vi "Element List to Scoring Cluster.vi"(11 "Array":cluster{"Name":string, "Value":string}[](array[cluster])) -> (0 "error out":errorcluster, 3 "output cluster":T1)   [LabVIEW 2013]
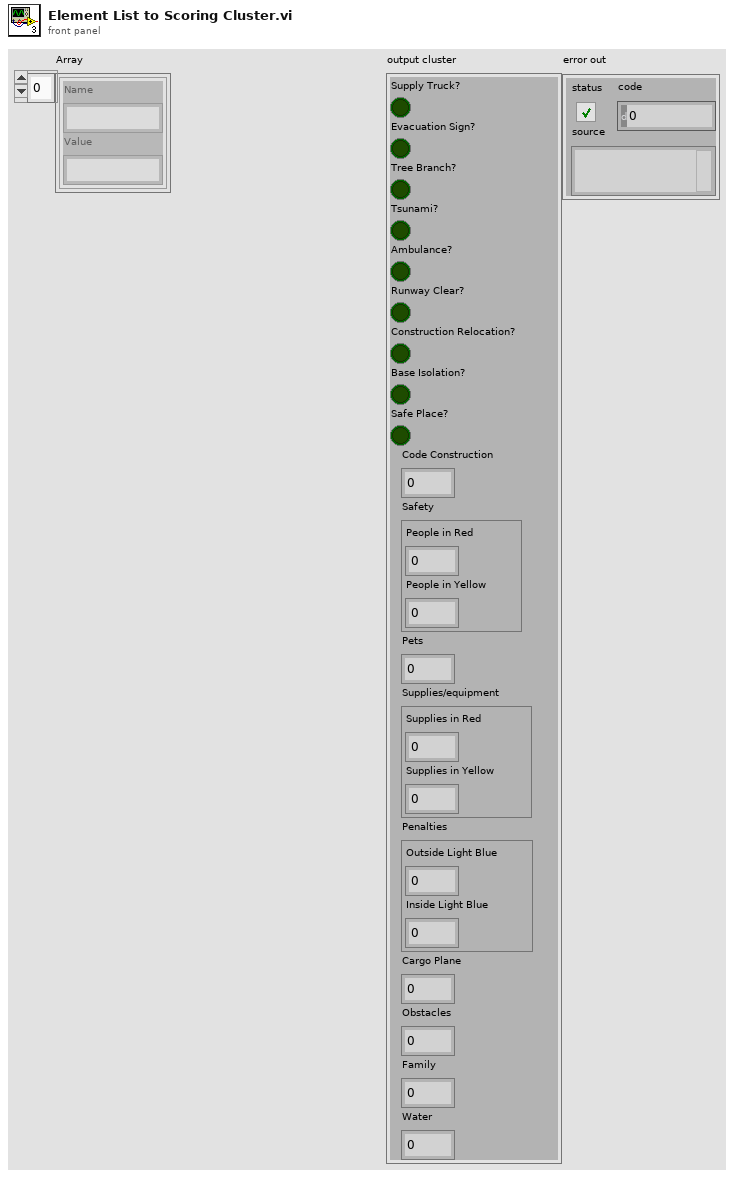
[diagram p1: front panel]
types:
  T1 = cluster{"Supply Truck?":bool, "Evacuation Sign?":bool, "Tree Branch?":bool, "Tsunami?":bool, "Ambulance?":bool, "Runway Clear?":bool, "Construction Relocation?":bool, "Base Isolation?":bool, "Safe Place?":bool, "Code Construction":dbl, "Safety":cluster{"People in Red":dbl, "People in Yellow":dbl}, "Pets":dbl, "Supplies/equipment":cluster{"Supplies in Red":dbl, "Supplies in Yellow":dbl}, "Penalties":cluster{"Outside Light Blue":dbl, "Inside Light Blue":dbl}, "Cargo Plane":u16, "Obstacles":u16, "Family":u16, "Water":dbl}
  T2 = cluster{"People in Red":dbl, "People in Yellow":dbl}
  T3 = cluster{"Outside Light Blue":dbl, "Inside Light Blue":dbl}
  T4 = cluster{"Supplies in Red":dbl, "Supplies in Yellow":dbl}
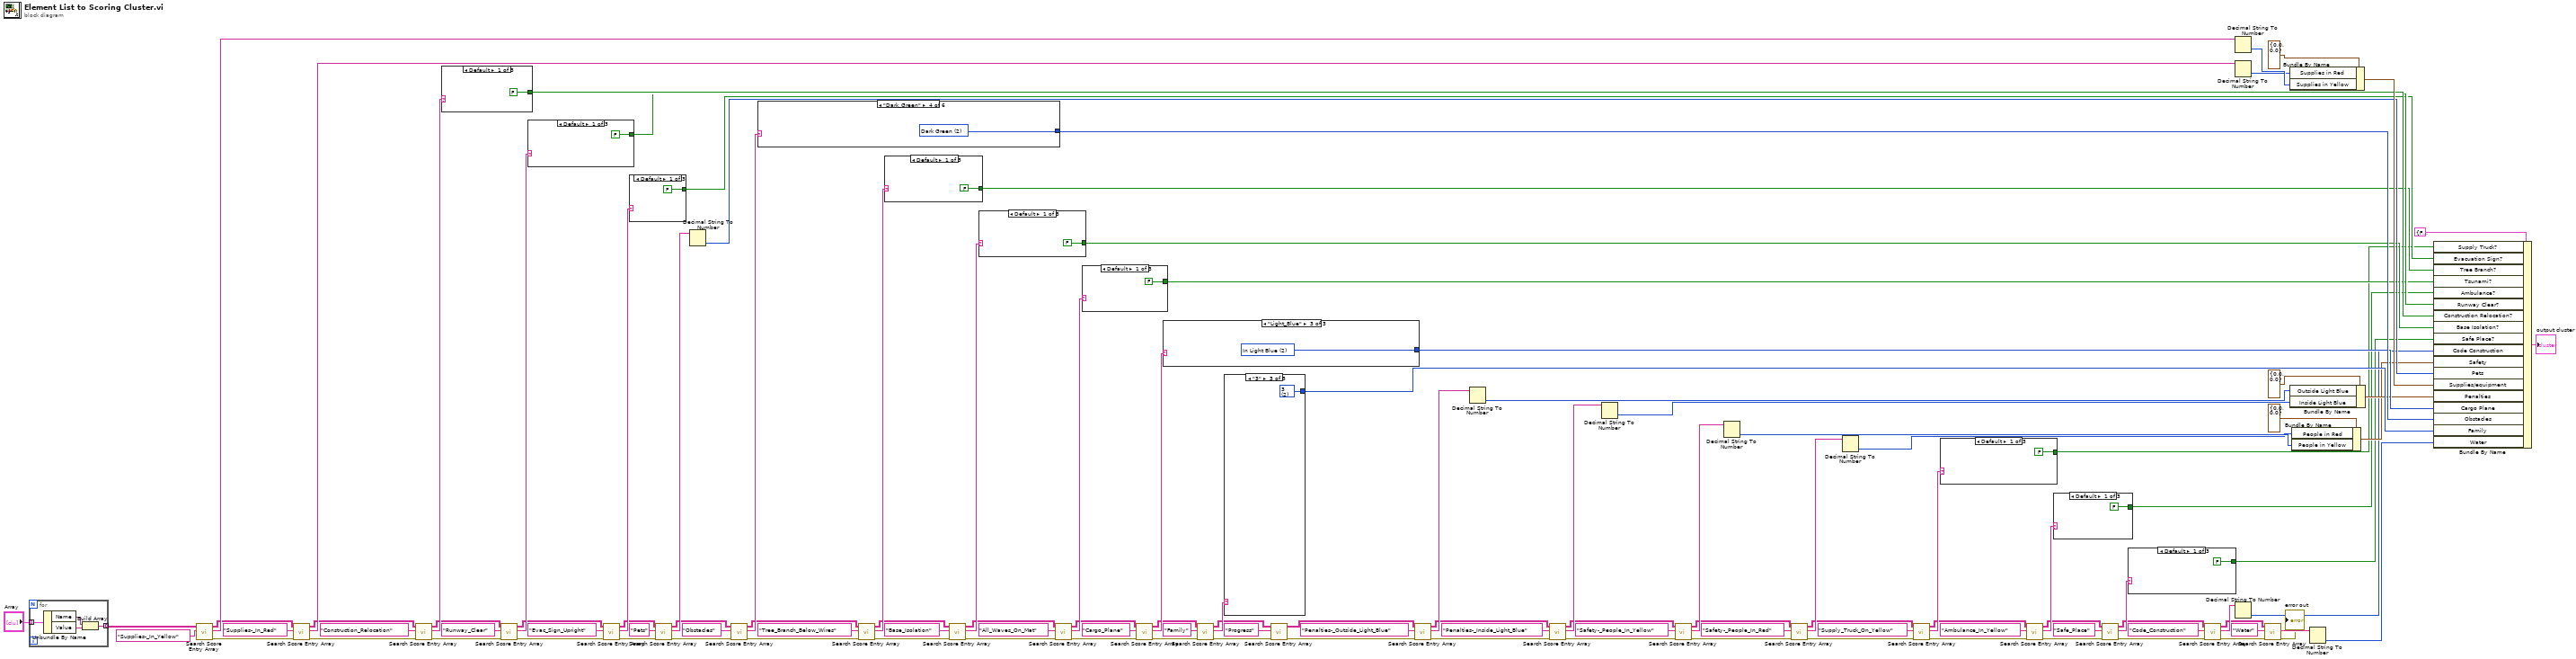
[diagram p0: block diagram]
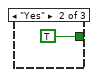
[diagram p2: hidden frame]
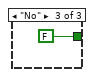
[diagram p3: hidden frame]
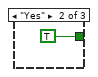
[diagram p4: hidden frame]
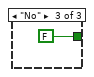
[diagram p5: hidden frame]
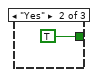
[diagram p6: hidden frame]
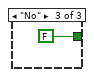
[diagram p7: hidden frame]
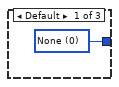
[diagram p8: hidden frame]
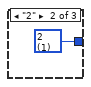
[diagram p9: hidden frame]
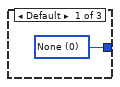
[diagram p10: hidden frame]
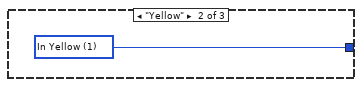
[diagram p11: hidden frame]
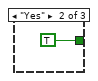
[diagram p12: hidden frame]
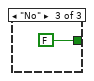
[diagram p13: hidden frame]
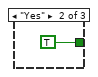
[diagram p14: hidden frame]
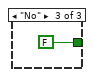
[diagram p15: hidden frame]
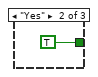
[diagram p16: hidden frame]
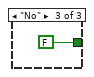
[diagram p17: hidden frame]
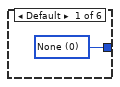
[diagram p18: hidden frame]
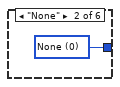
[diagram p19: hidden frame]
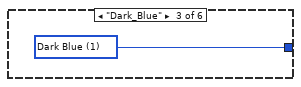
[diagram p20: hidden frame]
diagram:
  n1 = for {
    tunnel: "Array" -> [w121] mode=indexing
    tunnel: [w118] -> w115 mode=indexing
    n2 = Unbundle By Name(w121) -> ("Name"=w120:string, "Value"=w119:string)
    n3 = Build Array(w120, w119) -> (w118:string[])
  }
  n4 = call "Search Score Entry Array.vi"("Item Name"="Supplies-_In_Yellow", "Array"=w115) -> ("error out"=w108:errorcluster, "Value"=w113:string, "Array Out"=w109:string[][])  [unwired: 6 in, 1 out]
  n5 = call "Search Score Entry Array.vi"("error in (no error)"=w108, "Item Name"="Supplies-_In_Red", "Array"=w109) -> ("error out"=w103:errorcluster, "Value"=w106:string, "Array Out"=w104:string[][])  [unwired: 5 in, 1 out]
  n6 = call "Search Score Entry Array.vi"("error in (no error)"=w103, "Item Name"="Construction_Relocation", "Array"=w104) -> ("error out"=w98:errorcluster, "Value"=w101:string, "Array Out"=w99:string[][])  [unwired: 5 in, 1 out]
  n7 = case shown="Default" w101 {
    tunnel: [FALSE TRUE FALSE] -> w100
    frame Default {
    }
    frame "Yes" {
    }
    frame "No" {
    }
  }
  n8 = call "Search Score Entry Array.vi"("error in (no error)"=w98, "Item Name"="Runway_Clear", "Array"=w99) -> ("error out"=w93:errorcluster, "Value"=w96:string, "Array Out"=w94:string[][])  [unwired: 5 in, 1 out]
  n9 = case shown="Default" w96 {
    tunnel: [FALSE TRUE FALSE] -> w95
    frame Default {
    }
    frame "Yes" {
    }
    frame "No" {
    }
  }
  n10 = call "Search Score Entry Array.vi"("error in (no error)"=w93, "Item Name"="Evac_Sign_Upright", "Array"=w94) -> ("error out"=w88:errorcluster, "Value"=w91:string, "Array Out"=w89:string[][])  [unwired: 5 in, 1 out]
  n11 = case shown="Default" w91 {
    tunnel: [FALSE TRUE FALSE] -> w90
    frame Default {
    }
    frame "Yes" {
    }
    frame "No" {
    }
  }
  n12 = call "Search Score Entry Array.vi"("error in (no error)"=w88, "Item Name"="Pets", "Array"=w89) -> ("error out"=w83:errorcluster, "Value"=w86:string, "Array Out"=w84:string[][])  [unwired: 5 in, 1 out]
  n13 = Decimal String To Number(string=w86) -> (number=w85:i32)  [unwired: 2 in, 1 out]
  n14 = call "Search Score Entry Array.vi"("error in (no error)"=w83, "Item Name"="Obstacles", "Array"=w84) -> ("error out"=w79:errorcluster, "Value"=w81:string, "Array Out"=w78:string[][])  [unwired: 5 in, 1 out]
  n15 = case shown="\"Dark_Green\"" w81 {
    tunnel: [w131 w132 w133 w134 w135 w136] -> w80
    frame Default {
      w131 = u16 0 items=["None", "Dark Blue", "Dark Green", "Purple", "Red"] ("Obstacles")
    }
    frame "None" {
      w132 = u16 0 items=["None", "Dark Blue", "Dark Green", "Purple", "Red"] ("Obstacles")
    }
    frame "Dark_Blue" {
      w133 = u16 1 items=["None", "Dark Blue", "Dark Green", "Purple", "Red"] ("Obstacles")
    }
    frame "Dark_Green" {
      w134 = u16 2 items=["None", "Dark Blue", "Dark Green", "Purple", "Red"] ("Obstacles")
    }
    frame "Purple" {
      w135 = u16 3 items=["None", "Dark Blue", "Dark Green", "Purple", "Red"] ("Obstacles")
    }
    frame "Red" {
      w136 = u16 4 items=["None", "Dark Blue", "Dark Green", "Purple", "Red"] ("Obstacles")
    }
  }
  n16 = call "Search Score Entry Array.vi"("error in (no error)"=w79, "Item Name"="Tree_Branch_Below_Wires", "Array"=w78) -> ("error out"=w73:errorcluster, "Value"=w76:string, "Array Out"=w74:string[][])  [unwired: 5 in, 1 out]
  n17 = case shown="Default" w76 {
    tunnel: [FALSE TRUE FALSE] -> w75
    frame Default {
    }
    frame "Yes" {
    }
    frame "No" {
    }
  }
  n18 = call "Search Score Entry Array.vi"("error in (no error)"=w73, "Item Name"="Base_Isolation", "Array"=w74) -> ("error out"=w68:errorcluster, "Value"=w71:string, "Array Out"=w69:string[][])  [unwired: 5 in, 1 out]
  n19 = case shown="Default" w71 {
    tunnel: [FALSE TRUE FALSE] -> w70
    frame Default {
    }
    frame "Yes" {
    }
    frame "No" {
    }
  }
  n20 = call "Search Score Entry Array.vi"("error in (no error)"=w68, "Item Name"="All_Waves_On_Mat", "Array"=w69) -> ("error out"=w63:errorcluster, "Value"=w66:string, "Array Out"=w64:string[][])  [unwired: 5 in, 1 out]
  n21 = case shown="Default" w66 {
    tunnel: [FALSE TRUE FALSE] -> w65
    frame Default {
    }
    frame "Yes" {
    }
    frame "No" {
    }
  }
  n22 = call "Search Score Entry Array.vi"("error in (no error)"=w63, "Item Name"="Cargo_Plane", "Array"=w64) -> ("error out"=w58:errorcluster, "Value"=w61:string, "Array Out"=w59:string[][])  [unwired: 5 in, 1 out]
  n23 = case shown="\"Light_Blue\"" w61 {
    tunnel: [w146 w147 w148] -> w60
    frame Default {
      w146 = u16 0 items=["None", "In Yellow", "In Light Blue"] ("Cargo Plane")
    }
    frame "Yellow" {
      w147 = u16 1 items=["None", "In Yellow", "In Light Blue"] ("Cargo Plane")
    }
    frame "Light_Blue" {
      w148 = u16 2 items=["None", "In Yellow", "In Light Blue"] ("Cargo Plane")
    }
  }
  n24 = call "Search Score Entry Array.vi"("error in (no error)"=w58, "Item Name"="Family", "Array"=w59) -> ("error out"=w53:errorcluster, "Value"=w56:string, "Array Out"=w54:string[][])  [unwired: 5 in, 1 out]
  n25 = case shown="\"3\"" w56 {
    tunnel: [w149 w150 w151] -> w55
    frame Default {
      w149 = u16 0 items=["None", "2", "3"] ("Family")
    }
    frame "2" {
      w150 = u16 1 items=["None", "2", "3"] ("Family")
    }
    frame "3" {
      w151 = u16 2 items=["None", "2", "3"] ("Family")
    }
  }
  n26 = call "Search Score Entry Array.vi"("error in (no error)"=w53, "Item Name"="Progress", "Array"=w54) -> ("error out"=w50:errorcluster, "Array Out"=w51:string[][])  [unwired: 5 in, 2 out]
  n27 = call "Search Score Entry Array.vi"("error in (no error)"=w50, "Item Name"="Penalties-_Outside_Light_Blue", "Array"=w51) -> ("error out"=w43:errorcluster, "Value"=w46:string, "Array Out"=w44:string[][])  [unwired: 5 in, 1 out]
  n28 = Decimal String To Number(string=w46) -> (number=w45:i32)  [unwired: 2 in, 1 out]
  n29 = call "Search Score Entry Array.vi"("error in (no error)"=w43, "Item Name"="Penalties-_Inside_Light_Blue", "Array"=w44) -> ("error out"=w38:errorcluster, "Value"=w41:string, "Array Out"=w39:string[][])  [unwired: 5 in, 1 out]
  n30 = Decimal String To Number(string=w41) -> (number=w40:i32)  [unwired: 2 in, 1 out]
  n31 = call "Search Score Entry Array.vi"("error in (no error)"=w38, "Item Name"="Safety-_People_In_Yellow", "Array"=w39) -> ("error out"=w31:errorcluster, "Value"=w34:string, "Array Out"=w32:string[][])  [unwired: 5 in, 1 out]
  n32 = Decimal String To Number(string=w34) -> (number=w33:i32)  [unwired: 2 in, 1 out]
  n33 = call "Search Score Entry Array.vi"("error in (no error)"=w31, "Item Name"="Safety-_People_In_Red", "Array"=w32) -> ("error out"=w26:errorcluster, "Value"=w29:string, "Array Out"=w27:string[][])  [unwired: 5 in, 1 out]
  n34 = Decimal String To Number(string=w29) -> (number=w28:i32)  [unwired: 2 in, 1 out]
  n35 = call "Search Score Entry Array.vi"("error in (no error)"=w26, "Item Name"="Supply_Truck_On_Yellow", "Array"=w27) -> ("error out"=w21:errorcluster, "Value"=w24:string, "Array Out"=w22:string[][])  [unwired: 5 in, 1 out]
  n36 = case shown="Default" w24 {
    tunnel: [FALSE TRUE FALSE] -> w23
    frame Default {
    }
    frame "Yes" {
    }
    frame "No" {
    }
  }
  n37 = call "Search Score Entry Array.vi"("error in (no error)"=w21, "Item Name"="Ambulance_In_Yellow", "Array"=w22) -> ("error out"=w16:errorcluster, "Value"=w19:string, "Array Out"=w17:string[][])  [unwired: 5 in, 1 out]
  n38 = case shown="Default" w19 {
    tunnel: [FALSE TRUE FALSE] -> w18
    frame Default {
    }
    frame "Yes" {
    }
    frame "No" {
    }
  }
  n39 = call "Search Score Entry Array.vi"("error in (no error)"=w16, "Item Name"="Safe_Place", "Array"=w17) -> ("error out"=w11:errorcluster, "Value"=w14:string, "Array Out"=w12:string[][])  [unwired: 5 in, 1 out]
  n40 = case shown="Default" w14 {
    tunnel: [FALSE TRUE FALSE] -> w13
    frame Default {
    }
    frame "Yes" {
    }
    frame "No" {
    }
  }
  n41 = call "Search Score Entry Array.vi"("error in (no error)"=w11, "Item Name"="Code_Construction", "Array"=w12) -> ("error out"=w6:errorcluster, "Value"=w9:string, "Array Out"=w7:string[][])  [unwired: 5 in, 1 out]
  n42 = Decimal String To Number(string=w113) -> (number=w110:i32)  [unwired: 2 in, 1 out]
  n43 = Decimal String To Number(string=w106) -> (number=w105:i32)  [unwired: 2 in, 1 out]
  n44 = Decimal String To Number(string=w9) -> (number=w8:i32)  [unwired: 2 in, 1 out]
  n45 = call "Search Score Entry Array.vi"("error in (no error)"=w6, "Item Name"="Water", "Array"=w7) -> ("error out"=→"error out":errorcluster, "Value"=w4:string)  [unwired: 5 in, 2 out]
  n46 = Bundle By Name(cluster=T4 {"Supplies in Red"=0.0, "Supplies in Yellow"=0.0} ("Supplies/equipment"), "Supplies in Red"=w105, "Supplies in Yellow"=w110) -> (w111:T4)
  n47 = Bundle By Name(cluster=T3 {"Outside Light Blue"=0.0, "Inside Light Blue"=0.0} ("Penalties"), "Outside Light Blue"=w45, "Inside Light Blue"=w40) -> (w47:T3)
  n48 = Bundle By Name(cluster=T2 {"People in Red"=0.0, "People in Yellow"=0.0} ("Safety"), "People in Red"=w28, "People in Yellow"=w33) -> (w35:T2)
  n49 = Decimal String To Number(string=w4) -> (number=w3:i32)  [unwired: 2 in, 1 out]
  n50 = Bundle By Name(cluster=T1 {"Supply Truck?"=FALSE, "Evacuation Sign?"=FALSE, "Tree Branch?"=FALSE, "Tsunami?"=FALSE, "Ambulance?"=FALSE, "Runway Clear?"=FALSE, "Construction Relocation?"=FALSE, "Base Isolation?"=FALSE, "Safe Place?"=FALSE, "Code Construction"=0.0, "Safety"={"People in Red"=0.0, "People in Yellow"=0.0}, "Pets"=0.0, "Supplies/equipment"={"Supplies in Red"=0.0, "Supplies in Yellow"=0.0}, "Penalties"={"Outside Light Blue"=0.0, "Inside Light Blue"=0.0}, "Cargo Plane"=0, "Obstacles"=0, "Family"=0, "Water"=0.0} ("Scoring"), "Supply Truck?"=w23, "Evacuation Sign?"=w90, "Tree Branch?"=w75, "Tsunami?"=w65, "Ambulance?"=w18, "Runway Clear?"=w95, "Construction Relocation?"=w100, "Base Isolation?"=w70, "Safe Place?"=w13, "Code Construction"=w8, "Safety"=w35, "Pets"=w85, "Supplies/equipment"=w111, "Penalties"=w47, "Cargo Plane"=w60, "Obstacles"=w80, "Family"=w55, "Water"=w3) -> (→"output cluster":T1)
